vi "Send Connection Status.vi"(4 "Port":u16, 5 "Node ID":u32, 6 "Address":string, 7 "State":T1, 9 "TCPMessageAPI":refnum<class "TCPMessageAPI.lvclass">, 10 "Conn Handlers":refnum<queue>) -> ()   [LabVIEW 2020, in "Vecto.lvlib" / "TCPMessaging.lvclass"]
uses:
  TCPMessaging.lvclass
  TCPConnectionHandler/TCPConnectionHandler.lvclass
  TCPMessageService/TCPMessageAPI.lvclass
  Connection State.ctl
  Vecto.lvlib
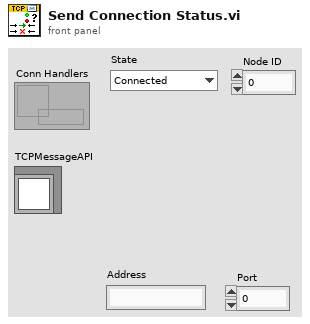
[diagram p1: front panel]
types:
  T1 = typedef "Vecto.lvlib/Connection State.ctl" = enum16{"Connected", "Disconnected"}
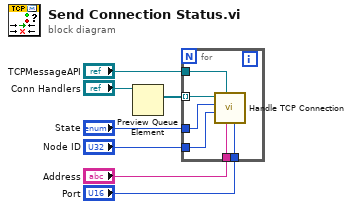
[diagram p0: block diagram]
diagram:
  n1 = Preview Queue Element(queue="Conn Handlers") -> (element=w6:refnum<class "TCPConnectionHandler.lvclass">[])  [unwired: 2 in, 3 out]
  n2 = for {
    tunnel: w6 -> [w13] mode=indexing
    tunnel: "TCPMessageAPI" -> [w12]
    tunnel: "Node ID" -> [w10]
    tunnel: "State" -> [w11]
    tunnel: "Address" -> [w9]
    tunnel: "Port" -> [w8]
    n3 = call-dynamic "Handle TCP Connection.vi"("Remote Port"=w8, "Remote Host"=w9, "TCPMessageAPI"=w12, "Node ID"=w10, "Connection State"=w11, "TCPConnectionHandler in"=w13) -> ()  [unwired: 4 in, 2 out]
  }
